vi "ReadFGV Err.vi"(8 "error in (no error)":errorcluster, 10 "0Cv/1ST":i32, 11 "LaserDetect01 in":refnum<class "LaserDetect01.lvclass">) -> (0 "error out":errorcluster, 3 "LaserDetect01 out":refnum<class "LaserDetect01.lvclass">)   [LabVIEW 2019, in "LaserDetect01.lvclass"]
uses:
  LaserDetect01.lvclass
  Ctrl/Auto Inspection Data Name.ctl
  Ctrl/Auto Inspection Station Name2.ctl
  e44b2bcd-d54f-4711-804d-ff8fbe0f93a7.vi
  <vilib>/JDP Science/JSONtext/JSON text to Variant.vi
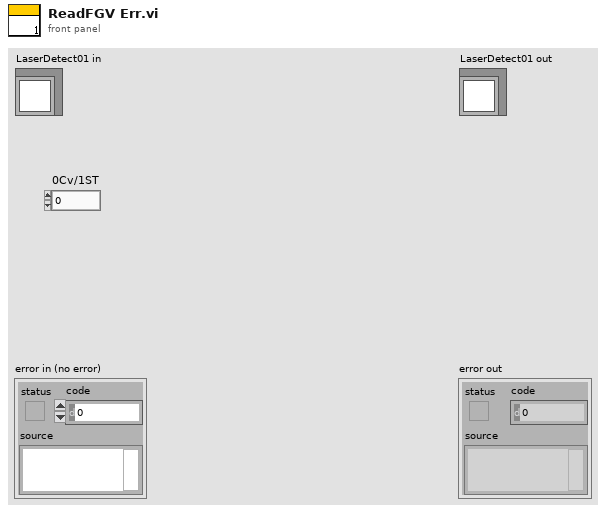
[diagram p1: front panel]
types:
  T1 = typedef "Auto Inspection Data Name.ctl" = enum16{"LocalRun", "ItemSN(TimeCode)", "CurrentAction", "Error", "Data", "OKNG", "電壓值", "電壓值判斷", "電流值", "電流值判斷", "Laser1 Data", "Laser2 Data", "Laser OKNG", "StationNO"}
  T2 = typedef "Auto Inspection Station Name2.ctl" = enum16{"S1Barcode", "S2Measure", "S3Measure", "S4Measure", "S5Measure", "S11_LaserCheck", "S8_Vision AI"}
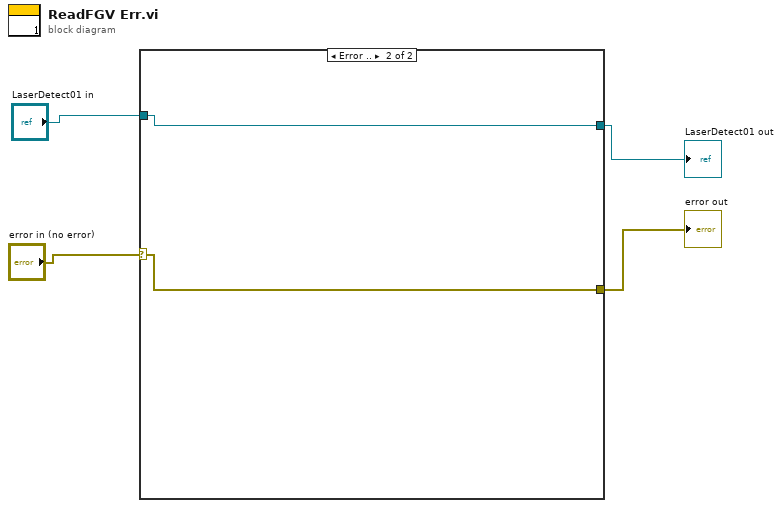
[diagram p0: block diagram]
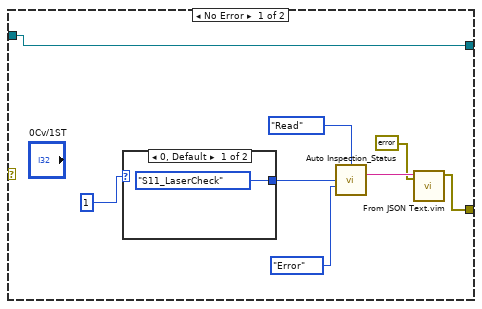
[diagram p2: hidden frame]
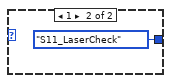
[diagram p3: hidden frame]
diagram:
  n1 = case shown="Error .." "error in (no error)" {
    selector: "error in (no error)" -> [_ w16]
    tunnel: [w7 w16] -> w3
    tunnel: "LaserDetect01 in" -> [w5 w15]
    tunnel: [w5 w15] -> w1
    frame No Error {
      n2 = case shown="0, Default" 1 {
        tunnel: [Auto_Inspection_Station_Name2."S11_LaserCheck" ("Station") Auto_Inspection_Station_Name2."S11_LaserCheck" ("Station")] -> w11
        frame 0, Default {
        }
        frame 1 {
        }
      }
      n3 = call "Auto Inspection_Status.vi"("Action"=enum16{"Initial", "Write", "Read"}."Read", "Station"=w11, "Data"=Auto_Inspection_Data_Name."Error") -> ("DataOut"=w9:string)  [unwired: 10 in, 2 out]
      n4 = call "From JSON Text.vim"("Data Type and Default Value"=errorcluster {"status"=FALSE, "code"=0, "source"=""} ("error constant"), "JSON"=w9) -> ("Data out"=w7:errorcluster)  [unwired: 8 in, 1 out]
    }
    frame Error {
    }
  }
  "error out" <- w3
  "LaserDetect01 out" <- w1
